vi "Angle Restrictions.vi"(4 "Min Forearm (degrees)":dbl, 5 "Min Backarm (degrees)":dbl, 6 "Max Forearm (degrees)":dbl, 7 "Max Backarm (degrees)":dbl, 10 "Forearm Angle 1":dbl, 11 "Backarm Angle 1":dbl) -> (2 "modified Forearm Angle 1":dbl, 3 "modified Backarm Angle 1":dbl)   [LabVIEW 2017]
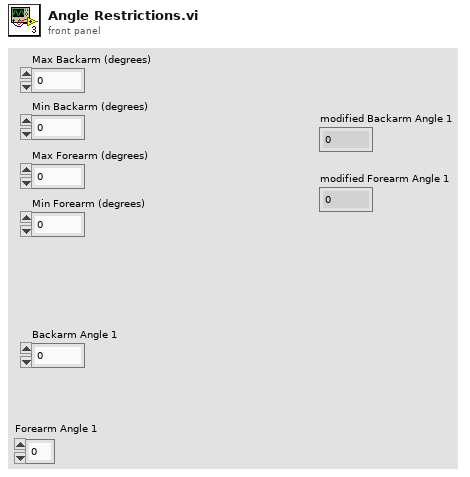
[diagram p1: front panel]
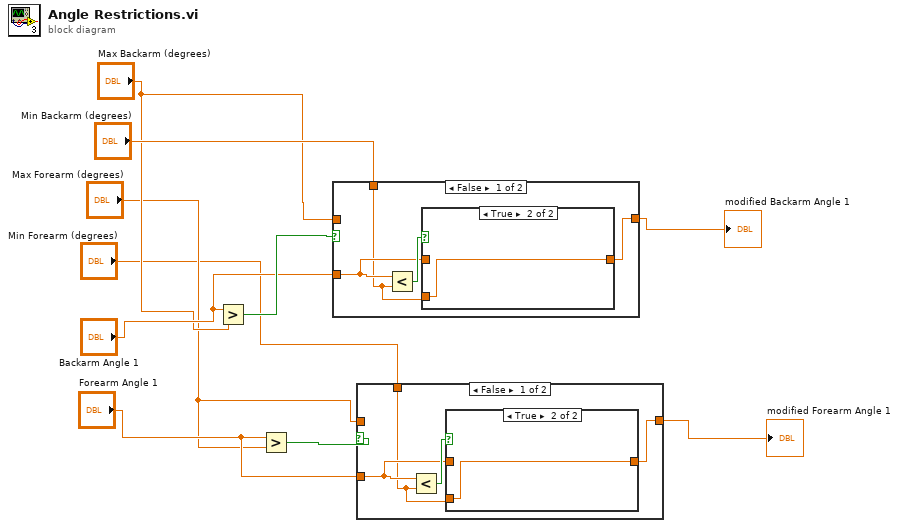
[diagram p0: block diagram]
diagram:
  n1 = Greater?(x="Backarm Angle 1", y="Max Backarm (degrees)") -> (0:w10:bool)
  n2 = Greater?(x="Forearm Angle 1", y="Max Forearm (degrees)") -> (0:w7:bool)
  n3 = case shown="False" w10 {
    tunnel: [w13 w17] -> w8
    tunnel: "Max Backarm (degrees)" -> [_ w17]
    tunnel: "Min Backarm (degrees)" -> [w11 _]
    tunnel: "Backarm Angle 1" -> [w12 _]
    frame False {
      n4 = Less?(x=w12, y=w11) -> (x < y?=w14:bool)
      n5 = case shown="True" w14 {
        tunnel: [w15 w16] -> w13
        tunnel: w12 -> [w15 _]
        tunnel: w11 -> [_ w16]
        frame False {
        }
        frame True {
        }
      }
    }
    frame True {
    }
  }
  "modified Backarm Angle 1" <- w8
  n6 = case shown="False" w7 {
    tunnel: [w20 w24] -> w6
    tunnel: "Max Forearm (degrees)" -> [_ w24]
    tunnel: "Min Forearm (degrees)" -> [w18 _]
    tunnel: "Forearm Angle 1" -> [w19 _]
    frame False {
      n7 = Less?(x=w19, y=w18) -> (x < y?=w21:bool)
      n8 = case shown="True" w21 {
        tunnel: [w22 w23] -> w20
        tunnel: w19 -> [w22 _]
        tunnel: w18 -> [_ w23]
        frame False {
        }
        frame True {
        }
      }
    }
    frame True {
    }
  }
  "modified Forearm Angle 1" <- w6
